vi "прямо.vi"() -> ()   [LabVIEW 2014]
uses:
  <vilib>/myRIO/Instrument Drivers/Utilities/Utilities.lvlib
  <vilib>/myRIO/Common/Instrument Driver Framework/myRIO v1.0/Encoder/typedefs/Encoder Count Direction Enum.ctl
panel:
  in  "left (A/DIO2 (Pin 15)) 2":bool
  in  "left (A/DIO2 (Pin 15))":bool
  in  "[ESC]":bool
  out "Counter Value":i32
  out "Counter Direction":T1
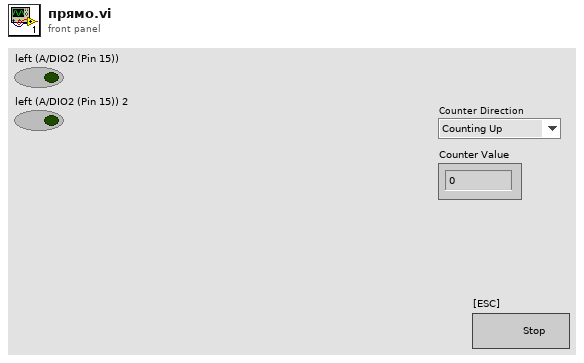
[diagram p1: front panel]
types:
  T1 = typedef "Encoder Count Direction Enum.ctl" = enum16{"Counting Up", "Counting Down"}
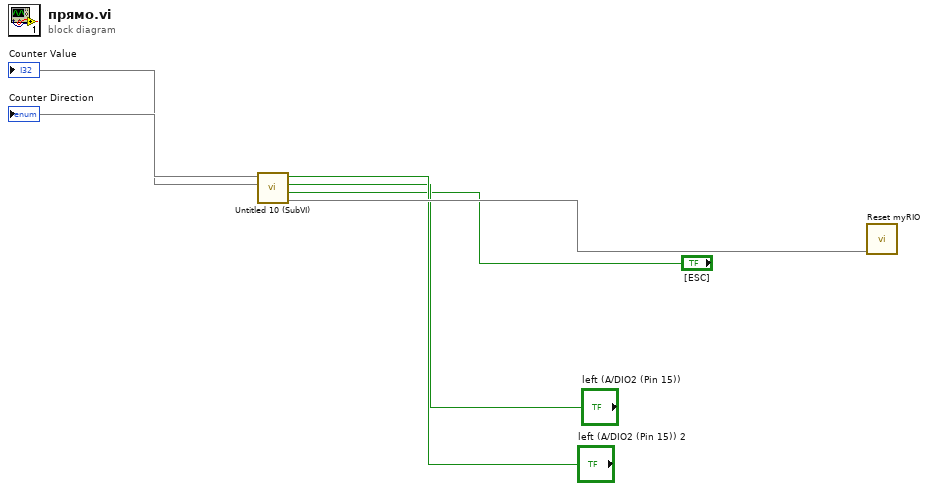
[diagram p0: block diagram]
diagram:
  n1 = call "Untitled 10 (SubVI).vi"(9:"[ESC]", 10:"left (A/DIO2 (Pin 15))", 11:"left (A/DIO2 (Pin 15)) 2") -> (0:w6, 2:→"Counter Value", 3:→"Counter Direction")  [unwired: 6 in]
  n2 = call <vilib>:"Reset myRIO.vi"("error in (no error)"=w6) -> ()  [unwired: 10 in, 1 out]
